vi "Execute.vi"(8 "error in":errorcluster, 11 "Change Temperature in":refnum<class "Change Temperature.lvclass">) -> (0 "error out":errorcluster, 1 "Next Step?":bool, 2 "MSG":string, 3 "Change Temperature out":refnum<class "Change Temperature.lvclass">)   [LabVIEW 2015, in "Change Temperature.lvclass"]
uses:
  Change Temperature.lvclass
  Reusable/Sequence/STEPS/LEAVES/Double/Switch DBL.lvclass/Switch DBL.ctl
  Change Temperature.lvclass/Change Temperature.ctl
  Reusable/Sequence/STEPS/LEAVES/Double/Read val.vi
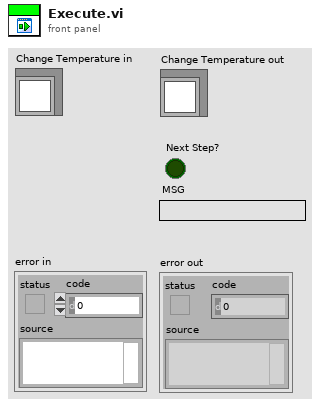
[diagram p1: front panel]
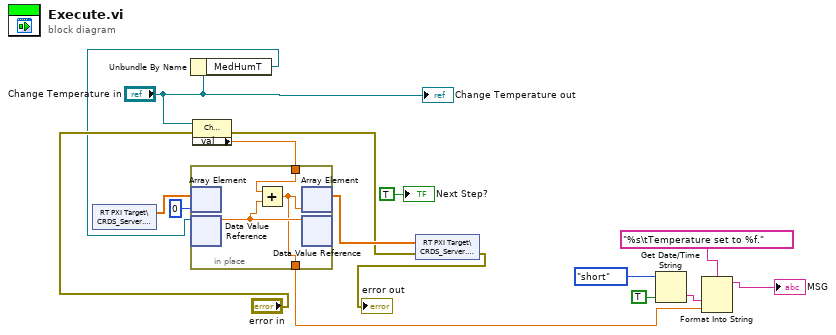
[diagram p0: block diagram]
diagram:
  n1 = shared-variable "RT PXI Target\\CRDS_Server.lvlib\\Tsp"() -> (w15:sgl[])  [unwired: 1 in, 1 out]
  n2 = Unbundle By Name("Change Temperature in") -> ("MedHumT"=w1:refnum<data-value>)
  n3 = property class="Change Temperature"(reference="Change Temperature in", error in="error in") -> (error out=w10:errorcluster, "val"=w13:dbl)  [unwired: 1 out]
  n4 = in-place {
    in-place-border: w13 -> [w19]
    in-place-border: [w17] -> w4
    n5 = in-place-array #1(w15, 0) -> ()  [unwired: 1 out]
    n6 = in-place-dvr #2(w1) -> (w18:dbl)  [unwired: 1 out]
    n7 = Add(x=w19, y=w18) -> (x+y=w17:dbl)
    n8 = in-place-array #1(w17) -> (w12:sgl[])  [unwired: 1 out]
    n9 = in-place-dvr #2(w18) -> ()  [unwired: 2 out]
  }
  n10 = shared-variable "RT PXI Target\\CRDS_Server.lvlib\\Tsp"(w12, error in=w10) -> (error out=→"error out":errorcluster)
  n11 = Get Date/Time String(date format (0)=enum16{"short", "long", "abbreviated"}."short", want seconds? (F)=TRUE) -> (time string=w6:string)  [unwired: 1 in, 1 out]
  n12 = Format Into String(format string="%s\tTemperature set to %f.", w6, w4) -> (resulting string=→"MSG":string)  [unwired: 2 in, 1 out]
  "Change Temperature out" <- "Change Temperature in"
  "Next Step?" <- TRUE ("Next Step?")
